vi "Check Handle Types.vi"() -> ()   [LabVIEW 2019]
uses:
  <vilib>/Utility/traverseref.llb/TRef TravTarget.ctl
  <vilib>/Utility/traverseref.llb/VI Scripting - Traverse.lvlib
  <vilib>/Utility/Data Type/NI_Data Type.lvlib
panel:
  out "Set":set{path}(c389)
  out "Checking/Updating...":path
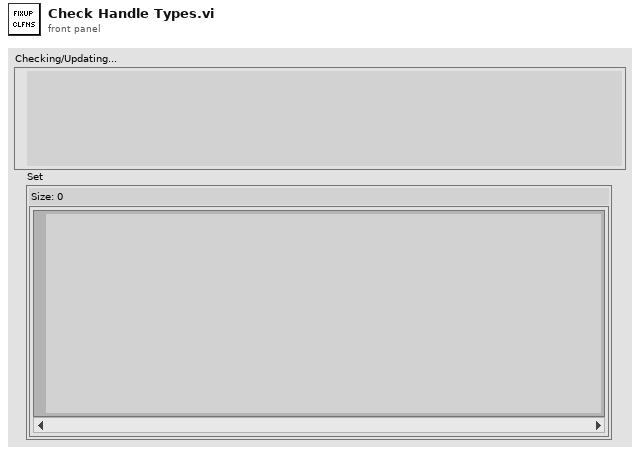
[diagram p1: front panel]
types:
  T1 = typedef "TRef TravTarget.ctl" = enum16{"FP", "BD", "Other"}
  T2 = cluster{"Parameter Name":string, "Num Dimensions":i32, "Parameter Type":enum16{"Numeric", "Array", "String", "Waveform", "Digital Waveform", "Digital Table", "ActiveX", "Any", "Instance Data Pointer", "Void"}, "Numeric Type":enum16{"I8", "I16", "I32", "I64", "U8", "U16", "U32", "U64", "SGL", "DBL", "PTR INT", "PTR UINT"}, "Param Passing":enum16{"By Value", "Pointer To Value"}, "Array Passing":enum16{"Array Data Pointer", "Array Handle", "Array Handle Pointer"}, "String Passing":enum16{"C String Pointer", "Pascal String Pointer", "String Handle", "String Handle Pointer"}, "Adapt Format":enum16{"By Value", "Pointer To Value"}, "ActiveX Types":enum16{"ActiveX Variant Pointer", "IDispatch* Pointer", "IUnknown* Pointer"}, "Const (unused)":bool, "Minimum Size":string}[]
  T3 = cluster{"Parameter Name":string, "Num Dimensions":i32, "Parameter Type":enum16{"Numeric", "Array", "String", "Waveform", "Digital Waveform", "Digital Table", "ActiveX", "Any", "Instance Data Pointer", "Void"}, "Numeric Type":enum16{"I8", "I16", "I32", "I64", "U8", "U16", "U32", "U64", "SGL", "DBL", "PTR INT", "PTR UINT"}, "Param Passing":enum16{"By Value", "Pointer To Value"}, "Array Passing":enum16{"Array Data Pointer", "Array Handle", "Array Handle Pointer"}, "String Passing":enum16{"C String Pointer", "Pascal String Pointer", "String Handle", "String Handle Pointer"}, "Adapt Format":enum16{"By Value", "Pointer To Value"}, "ActiveX Types":enum16{"ActiveX Variant Pointer", "IDispatch* Pointer", "IUnknown* Pointer"}, "Const (unused)":bool, "Minimum Size":string}
  T4 = enum16{"Numeric", "Array", "String", "Waveform", "Digital Waveform", "Digital Table", "ActiveX", "Any", "Instance Data Pointer", "Void"}
  T5 = typedef "NI_Data Type.lvlib/Data Type.ctl" = enum8{"Invalid Type", "Void", "I8", "I16", "I32", "I64", "U8", "U16", "U32", "U64", "Single Float", "Double Float", "Extended Float", "Single Complex", "Double Complex", "Extended Complex", "Enum U8", "Enum U16", "Enum U32", "Enum U64", "Single Float With Unit", "Double Float With Unit", "Extended Float With Unit", "Single Complex with Unit", "Double Complex with Unit", "Extended Complex with Unit", "Boolean", "String", "Path", "Picture", "Tag", "Array", "Cluster", "Variant", "LV Variant", "Waveform", "Timestamp", "Digital Waveform", "Digital Data", "ExpressData", "Refnum", "External Data", "VI", "Poly VI", "LabVIEW Class Instance", "Fixed Point", "Set Collection", "Map Collection"}
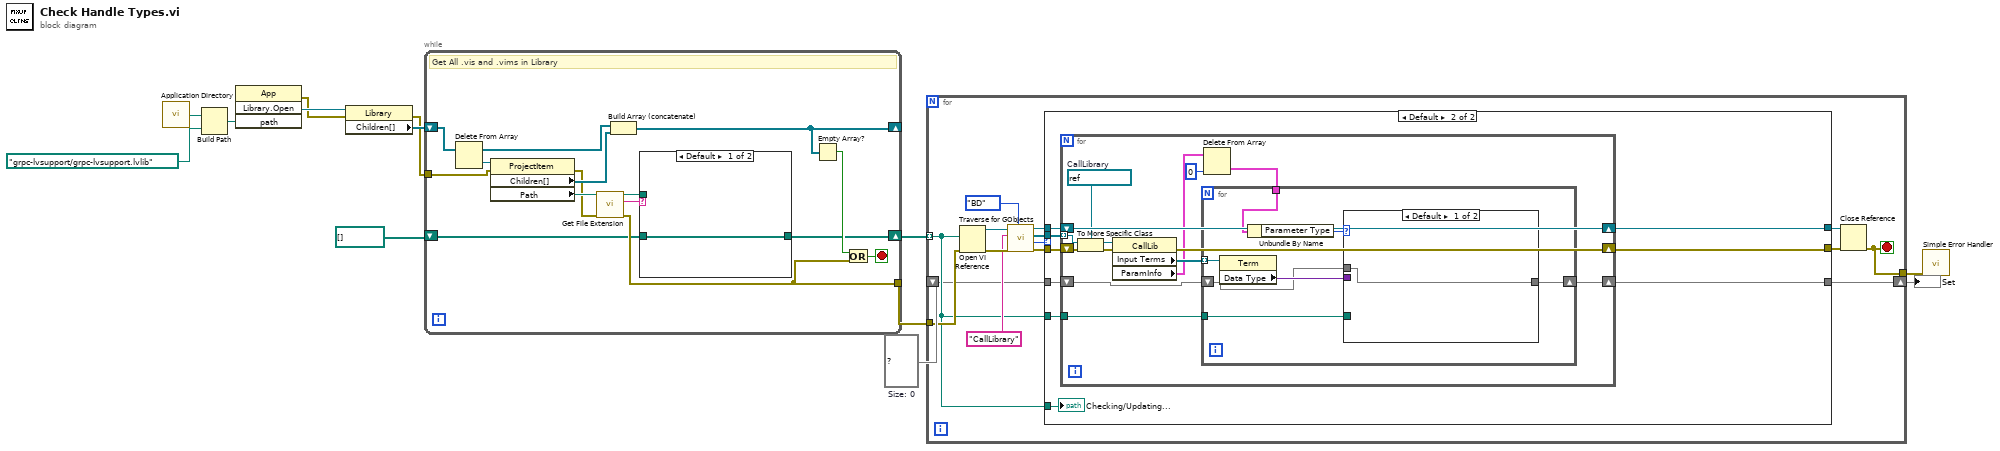
[diagram p0: block diagram]
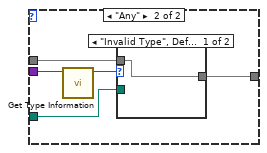
[diagram p3: hidden frame]
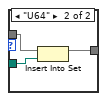
[diagram p4: hidden frame]
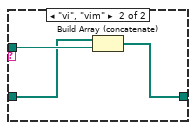
[diagram p5: hidden frame]
diagram:
  w2 = set{path} {}  # Size: 0
  n1 = call <vilib>:"Application Directory.vi"() -> ("Application Directory"=w13:path)
  n2 = Build Path(base path=w13, name or relative path=path "grpc-lvsupport/grpc-lvsupport.lvlib") -> (appended path=w11:path)
  n3 = invoke class="App" method="Library.Open"("path"=w11) -> (error out=w8:errorcluster, "Open Library"=w10:refnum<vi>)  [unwired: 3 in, 2 out]
  n4 = property class="Library"(reference=w10, error in=w8) -> (error out=w7:errorcluster, "Children[]"=w9:refnum<vi>[])  [unwired: 1 out]
  n5 = while {
    shift-right: [w24] -> _
    shift-left: w9 -> [w28]
    tunnel: w7 -> [w19]
    tunnel: [w16] -> w4
    shift-right: [w14] -> w5
    shift-left: path[] [] ("appended array") -> [w15]
    stop <- w17 stop-if-true
    # "Get All .vis and .vims in Library"
    n6 = Delete From Array(array=w28) -> (deleted portion=w27:refnum<vi>, array with subset deleted=w26:refnum<vi>[])  [unwired: 2 in]
    n7 = property class="ProjectItem"(reference=w27, error in=w19) -> (error out=w18:errorcluster, "Children[]"=w25:refnum<vi>[], "Path"=w22:path)  [unwired: 1 out]
    n8 = call <vilib>:"Get File Extension.vi"("error in (no error)"=w18, "file"=w22) -> ("error out"=w16:errorcluster, "lowercase file extension"=w21:string, "dup file"=w20:path)  [unwired: 5 in, 2 out]
    n9 = Build Array (concatenate)(w26, w25) -> (w24:refnum<vi>[])
    n10 = case shown="Default" w21 {
      tunnel: w20 -> [_ w32]
      tunnel: w15 -> [w29 w31]
      tunnel: [w29 w30] -> w14
      frame Default {
      }
      frame "vi", "vim" {
        n11 = Build Array (concatenate)(w31, w32) -> (w30:path[])
      }
    }
    n12 = Empty Array?(array=w24) -> (empty?=w23:bool)
    n13 = Or(x=w23, y=w16) -> (x .or. y?=w17:bool)
  }
  n14 = for {
    tunnel: w5 -> [w35] mode=indexing
    tunnel: w4 -> [w47]
    tunnel: [w36] -> w3
    shift-right: [w34] -> w1
    shift-left: w2 -> [w33]
    stop <- w36 stop-if-true
    n15 = Open VI Reference(vi path=w35, error in (no error)=w47) -> (vi reference=w46:refnum<vi>, error out=w45:errorcluster)  [unwired: 4 in]
    n16 = call <vilib>:"Traverse for GObjects.vi"("Traverse Target"=TRef_TravTarget."BD", "error in (no error)"=w45, "Class Name"="CallLibrary", "VI Refnum"=w46) -> ("error out"=w42:errorcluster, "# of Refs"=w39:i32, "References"=w43:refnum<vi>[], "dup VI Refnum"=w40:refnum<vi>)  [unwired: 4 in]
    n17 = case shown="Default" w39 {
      tunnel: w43 -> [_ w59]
      tunnel: w42 -> [w49 w58]
      tunnel: w40 -> [w50 w57]
      tunnel: [w50 w56] -> w37
      tunnel: [w49 w55] -> w38
      tunnel: w35 -> [_ w54]
      tunnel: w35 -> [_ w53]
      tunnel: [w48 w52] -> w34
      tunnel: w33 -> [w48 w51]
      frame ..0 {
      }
      frame Default {
        n18 = for {
          tunnel: w59 -> [w73] mode=indexing
          shift-right: [w68] -> w56
          shift-left: w57 -> [w68]
          shift-right: [w69] -> w55
          shift-left: w58 -> [w72]
          tunnel: w53 -> [w62]
          shift-right: [w61] -> w52
          shift-left: w51 -> [w60]
          w67 = refnum<vi> refnum  # CallLibrary
          n19 = To More Specific Class(target class=w67, reference=w73, error in=w72) -> (specific class reference=w70:refnum<vi>, error out=w71:errorcluster)
          n20 = property class="CallLib"(reference=w70, error in=w71) -> (error out=w69:errorcluster, "Input Terms"=w66:refnum<vi>[], "ParamInfo"=w65:T2)  [unwired: 1 out]
          n21 = Delete From Array(array=w65, index=0) -> (deleted portion=w63:T3)  [unwired: 1 in, 1 out]
          n22 = for {
            tunnel: w66 -> [w80] mode=indexing
            tunnel: w63 -> [w79]
            tunnel: w62 -> [w76]
            shift-right: [w75] -> w61
            shift-left: w60 -> [w74]
            n23 = property class="Term"(reference=w80) -> ("Data Type"=w77:variant)  [unwired: 1 in, 2 out]
            n24 = Unbundle By Name(w79) -> ("Parameter Type"=w78:T4)
            n25 = case shown="Default" w78 {
              tunnel: w77 -> [_ w86]
              tunnel: w76 -> [_ w84]
              tunnel: [w81 w83] -> w75
              tunnel: w74 -> [w81 w82]
              frame Default {
              }
              frame "Any" {
                n26 = call <vilib>:"Get Type Information.vi"("variant"=w86) -> ("type"=w85:T5)  [unwired: 6 in, 4 out]
                n27 = case shown="\"Invalid Type\", Default" w85 {
                  tunnel: w84 -> [_ w90]
                  tunnel: [w87 w89] -> w83
                  tunnel: w82 -> [w87 w88]
                  frame "Invalid Type", Default {
                  }
                  frame "U64" {
                    n28 = Insert Into Set(10:w90, 11:w88) -> (3:w89:set{path})  [unwired: 1 out]
                  }
                }
              }
            }
          }
        }
        "Checking/Updating..." <- w54
      }
    }
    n29 = Close Reference(reference=w37, error in (no error)=w38) -> (error out=w36:errorcluster)
  }
  "Set" <- w1
  n30 = call <vilib>:"Simple Error Handler.vi"("error in (no error)"=w3) -> ()  [unwired: 4 in, 5 out]
